vi "MTM2_putSample_tangentForcesMeasured.vi"(8 "error in (no error)":errorcluster, 11 "tangentForcesMeasured_Ctl":T1) -> (0 "error out":errorcluster, 2 "function return":i32, 3 "tangentForcesMeasured_Ctl out":T1)   [LabVIEW 2018, in "SALLV_MTM2.lvlib"]
doc: "int MTM2_shm_putSample_tangentForcesMeasuredLV(MTM2_tangentForcesMeasuredLV *tangentForcesMeasured_Ctl );"
uses:
  SALLV_MTM2.lvlib
  DataTypes/tangentForcesMeasured.ctl
  SALLV_MTM2.so
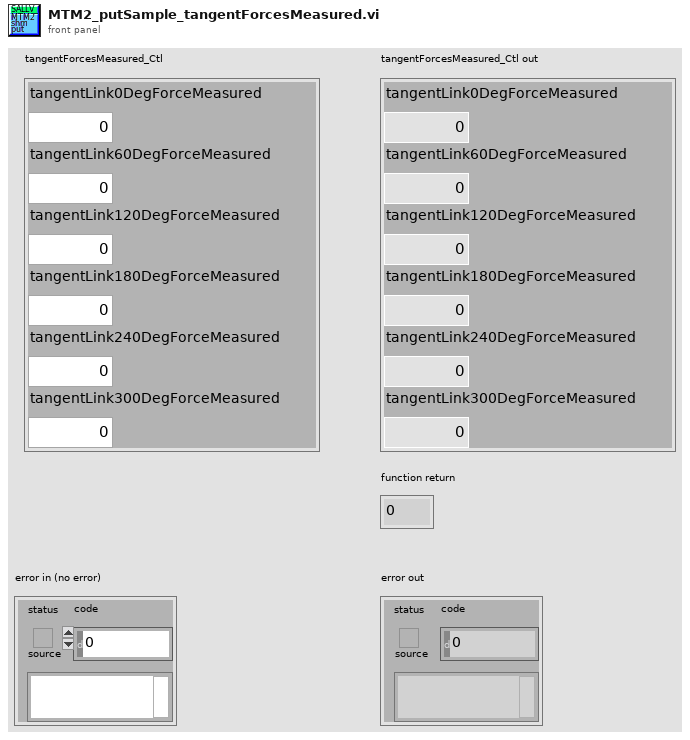
[diagram p1: front panel]
types:
  T1 = typedef "SALLV_MTM2.lvlib/tangentForcesMeasured.ctl" = cluster{"tangentLink0DegForceMeasured":dbl, "tangentLink60DegForceMeasured":dbl, "tangentLink120DegForceMeasured":dbl, "tangentLink180DegForceMeasured":dbl, "tangentLink240DegForceMeasured":dbl, "tangentLink300DegForceMeasured":dbl}
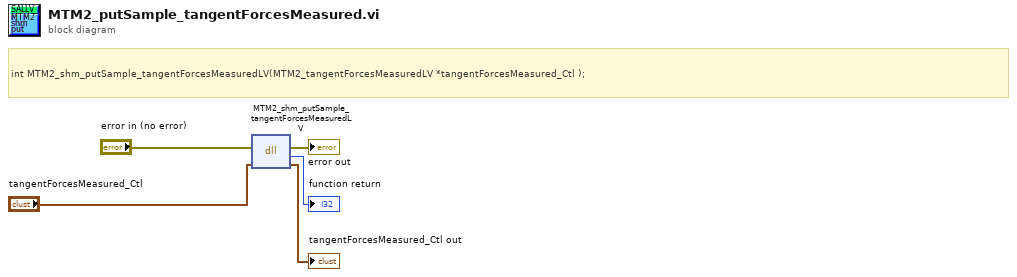
[diagram p0: block diagram]
diagram:
  # "int MTM2_shm_putSample_tangentForcesMeasuredLV(MTM2_tangentForcesMeasuredLV *tangentForcesMeasured_Ctl );"
  n1 = dll-call lib="home/ttsai/Document/salApiMTM2/SALLV_MTM2/SALLV_MTM2.*" fn="MTM2_shm_putSample_tangentForcesMeasuredLV"(error in="error in (no error)", "tangentForcesMeasured_Ctl"="tangentForcesMeasured_Ctl") -> (error out=→"error out":errorcluster, →"function return":i32, "tangentForcesMeasured_Ctl"=→"tangentForcesMeasured_Ctl out":T1)  [unwired: 2 in, 1 out]
